vi "Write AnchorY.vi"(2 "error in (no error)":errorcluster, 3 "AnchorY":dbl, 4 "Anchor in":refnum<class "Anchor.lvclass">) -> (0 "error out":errorcluster, 1 "Anchor out":refnum<class "Anchor.lvclass">)   [LabVIEW 2014, in "Anchor.lvclass"]
uses:
  Anchor.lvclass
  Anchor.lvclass/Anchor.ctl
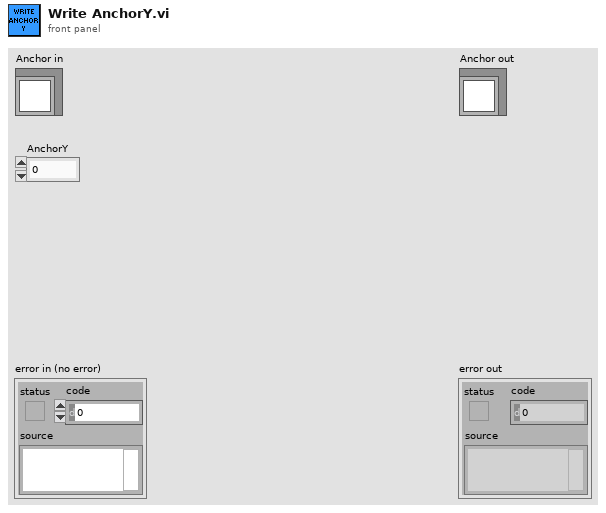
[diagram p1: front panel]
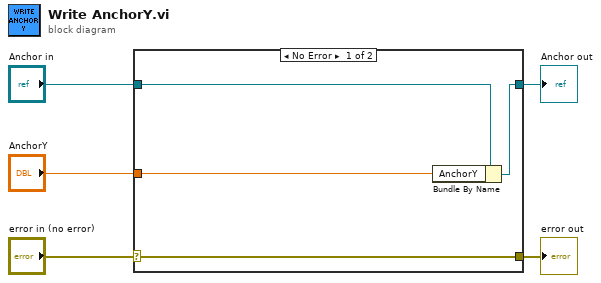
[diagram p0: block diagram]
diagram:
  n1 = case shown="No Error" "error in (no error)" {
    selector: "error in (no error)" -> [w9 w10]
    tunnel: [w9 w10] -> w4
    tunnel: [w7 w11] -> w2
    tunnel: "Anchor in" -> [w8 w11]
    tunnel: "AnchorY" -> [w6 _]
    frame No Error {
      n2 = Bundle By Name(cluster=w8, "AnchorY"=w6) -> (w7:refnum<class "Anchor.lvclass">)
    }
    frame Error {
    }
  }
  "error out" <- w4
  "Anchor out" <- w2
